vi "Generator DC Sweep Manager.vi"(8 "error in (no error)":errorcluster, 10 "sweep index":i32=-1, 11 "LockinDAQ":refnum<class "LockinDAQ.lvclass">) -> (0 "error out":errorcluster, 1 "Start (V)":dbl[](array[numeric]), 2 "End (V)":dbl[](array[numeric]), 3 "LockinDAQ out":refnum<class "LockinDAQ.lvclass">)   [LabVIEW 2016, in "LockinDAQ.lvclass"]
uses:
  LockinDAQ.lvclass
  LockinDAQ.lvclass/LockinDAQ.ctl
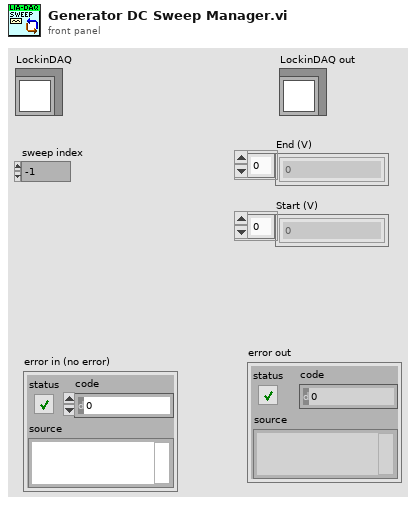
[diagram p1: front panel]
types:
  T1 = typedef "LockinDAQ.lvclass/AO-cluster.ctl" = cluster{"Ch":i32[], "Amp (V)":dbl[], "DC (V)":dbl[], "f (Hz)":dbl[], "Phase (°)":dbl[], "Function":T2[], "Sweep?":bool[]}
  T2 = typedef "LockinDAQ.lvclass/Function-enum.ctl" = enum16{"Sine", "Triangle", "Square", "Sawtooth"}
  T3 = typedef "LockinDAQ.lvclass/Sweep Configuration--Cluster.ctl" = cluster{"Sweep Type":enum16{"sweepLockin", "sweepIV"}, "Sweep Lockin Time (s)":dbl, "Sweep IV Step (V)":dbl, "Initial Wait Time (s)":dbl, "Sweep Channel":i32[], "Sweep Start (V)":dbl[], "Sweep End (V)":dbl[], "Return to Start":bool}
  T4 = typedef "LockinDAQ.lvclass/Sampling.ctl" = cluster{"Fs":dbl, "#s":i32}
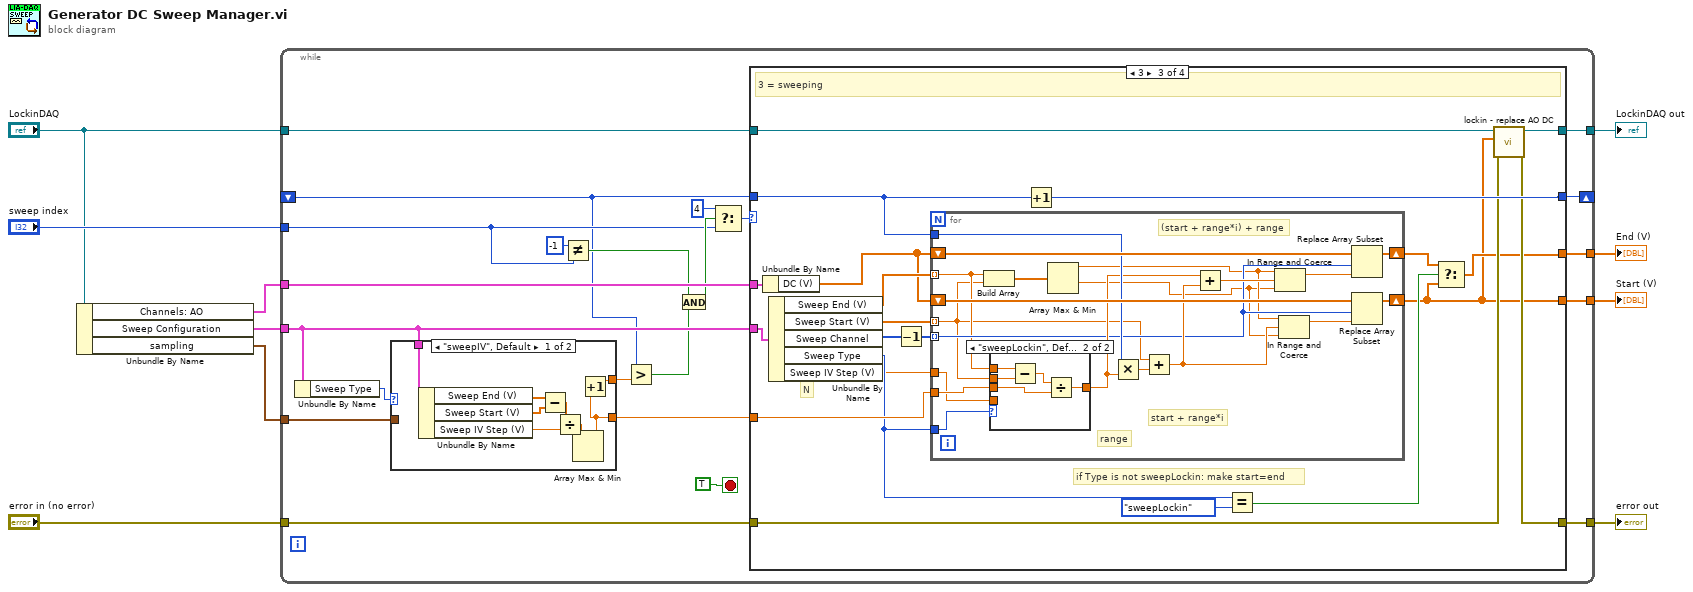
[diagram p0: block diagram]
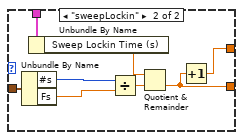
[diagram p2: hidden frame]
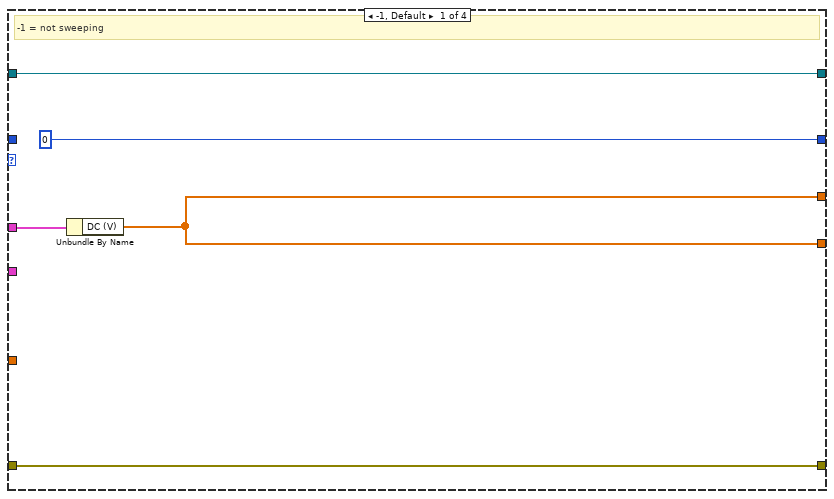
[diagram p3: hidden frame]
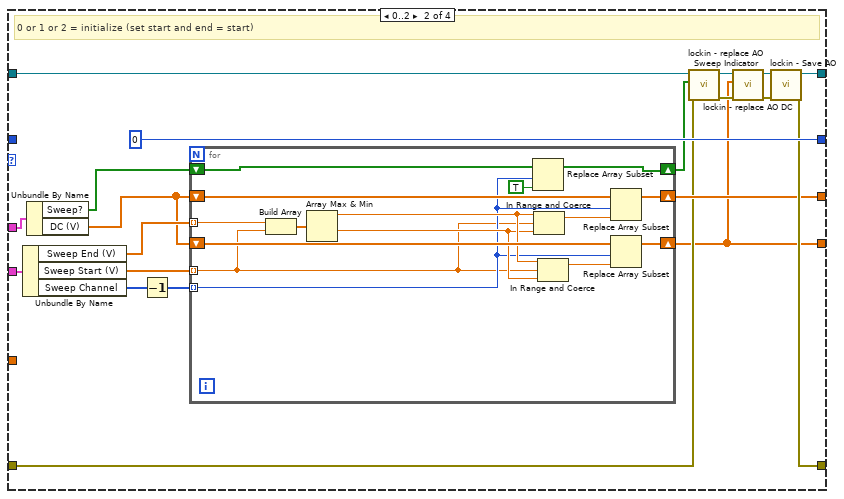
[diagram p4: hidden frame]
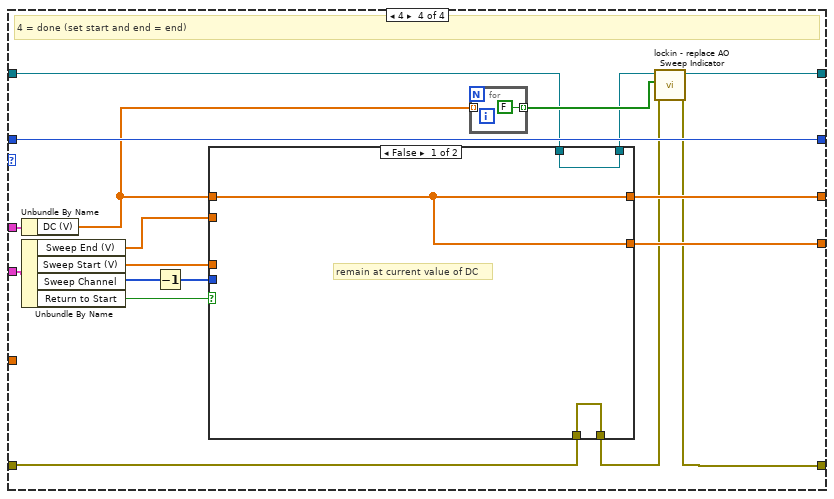
[diagram p6: hidden frame]
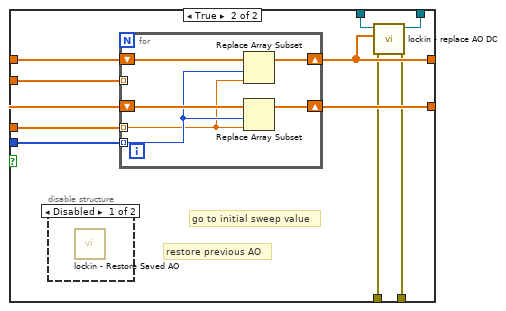
[diagram p7: hidden frame]
diagram:
  n1 = Unbundle By Name("LockinDAQ") -> ("Channels: AO"=w6:T1, "Sweep Configuration"=w7:T3, "sampling"=w8:T4)
  n2 = while {
    tunnel: w6 -> [w32]
    tunnel: [w17] -> w9
    tunnel: [w31] -> w10
    tunnel: w7 -> [w15]
    tunnel: "sweep index" -> [w16]
    tunnel: w8 -> [w28]
    shift-right: [w30] -> _
    shift-left: _ -> [w12]
    tunnel: [w21] -> w4
    tunnel: "LockinDAQ" -> [w20]
    tunnel: "error in (no error)" -> [w19]
    tunnel: [w18] -> w1
    stop <- TRUE stop-if-true
    n3 = Unbundle By Name(w15) -> ("Sweep Type"=w14:enum16{"sweepLockin", "sweepIV"})
    n4 = case shown="\"sweepIV\", Default" w14 {
      tunnel: w28 -> [_ w44]
      tunnel: [w34 w43] -> w25
      tunnel: w15 -> [w40 w42]
      tunnel: [w33 w41] -> w13
      frame "sweepIV", Default {
        n5 = Unbundle By Name(w40) -> ("Sweep End (V)"=w39:dbl[], "Sweep Start (V)"=w38:dbl[], "Sweep IV Step (V)"=w36:dbl)
        n6 = Subtract(x=w39, y=w38) -> (x-y=w37:dbl[])
        n7 = Divide(x=w37, y=w36) -> (x/y=w35:dbl[])
        n8 = Array Max & Min(array=w35) -> (max value=w34:dbl)  [unwired: 3 out]
        n9 = Increment(x=w34) -> (x+1=w33:dbl)
      }
      frame "sweepLockin" {
        n10 = Unbundle By Name(w44) -> ("#s"=w45:i32, "Fs"=w48:dbl)
        n11 = Unbundle By Name(w42) -> ("Sweep Lockin Time (s)"=w47:dbl)
        n12 = Divide(x=w45, y=w48) -> (x/y=w46:dbl)
        n13 = Quotient & Remainder(x=w47, y=w46) -> (floor(x/y)=w43:dbl)  [unwired: 1 out]
        n14 = Increment(x=w43) -> (x+1=w41:dbl)
      }
    }
    n15 = Not Equal?(x=-1, y=w16) -> (x != y?=w22:bool)
    n16 = Greater?(x=w12, y=w13) -> (0:w11:bool)
    n17 = And(x=w22, y=w11) -> (x .and. y?=w23:bool)
    n18 = Select(t=4, s=w23, f=w16) -> (s? t:f=w26:i32)
    n19 = case shown="3" w26 {
      tunnel: w32 -> [w53 w73 w109 w153]
      tunnel: [w52 w54 w91 w151] -> w31
      tunnel: w15 -> [_ w69 w105 w148]
      tunnel: [0 0 w101 w146] -> w30
      tunnel: w12 -> [_ _ w102 w146]
      tunnel: w25 -> [_ _ w100 _]
      tunnel: [w50 w65 w96 w137] -> w21
      tunnel: w20 -> [w50 w61 w98 w141]
      tunnel: w19 -> [w49 w57 w99 w139]
      tunnel: [w49 w64 w97 w136] -> w18
      tunnel: [w52 w62 w92 w145] -> w17
      frame -1, Default {
        # "-1 = not sweeping"
        n20 = Unbundle By Name(w53) -> ("DC (V)"=w52:dbl[])
      }
      frame 0..2 {
        # "0 or 1 or 2 = initialize (set start and end = start)"
        n21 = Unbundle By Name(w69) -> ("Sweep End (V)"=w70:dbl[], "Sweep Start (V)"=w71:dbl[], "Sweep Channel"=w72:i32[])
        n22 = Unbundle By Name(w73) -> ("Sweep?"=w59:bool[], "DC (V)"=w67:dbl[])
        n23 = Decrement(x=w72) -> (x-1=w68:i32[])
        n24 = for {
          shift-right: [w87] -> w62
          shift-left: w67 -> [w88]
          shift-right: [w85] -> w54
          shift-left: w67 -> [w86]
          tunnel: w71 -> [w74] mode=indexing
          tunnel: w70 -> [w81] mode=indexing
          tunnel: w68 -> [w76] mode=indexing
          shift-right: [w77] -> w55
          shift-left: w59 -> [w78]
          n25 = Build Array(w81, w74) -> (w82:dbl[])
          n26 = Array Max & Min(array=w82) -> (max value=w80:dbl, min value=w79:dbl)  [unwired: 2 out]
          n27 = Replace Array Subset(array=w78, new element=TRUE ("new element/subarray"), index=w76) -> (w77:bool[])
          n28 = In Range and Coerce(upper limit=w80, x=w74, lower limit=w79) -> (coerced(x)=w84:dbl)  [unwired: 1 out]
          n29 = In Range and Coerce(upper limit=w80, x=w74, lower limit=w79) -> (coerced(x)=w83:dbl)  [unwired: 1 out]
          n30 = Replace Array Subset(array=w88, new element=w84, index=w76) -> (w87:dbl[])
          n31 = Replace Array Subset(array=w86, new element=w83, index=w76) -> (w85:dbl[])
        }
        n32 = call "lockin - replace AO Sweep Indicator.vi"("error in (no error)"=w57, "Channels: AO.Sweep?"=w55, "LockinDAQ"=w61) -> ("error out"=w58:errorcluster, "LockinDAQ out"=w60:refnum<class "LockinDAQ.lvclass">)  [unwired: 7 in]
        n33 = call "lockin - replace AO DC.vi"("error in (no error)"=w58, "AO.DC (V)"=w54, "LockinDAQ"=w60) -> ("error out"=w56:errorcluster, "LockinDAQ out"=w63:refnum<class "LockinDAQ.lvclass">)  [unwired: 7 in]
        n34 = call "lockin - Save AO.vi"("error in (no error)"=w56, "LockinDAQ"=w63) -> ("error out"=w64:errorcluster, "LockinDAQ out"=w65:refnum<class "LockinDAQ.lvclass">)  [unwired: 8 in]
      }
      frame 3 {
        # "if Type is not sweepLockin: make start=end"
        # "N"
        # "3 = sweeping"
        n35 = Unbundle By Name(w109) -> ("DC (V)"=w103:dbl[])
        n36 = Unbundle By Name(w105) -> ("Sweep End (V)"=w106:dbl[], "Sweep Start (V)"=w107:dbl[], "Sweep Channel"=w108:i32[], "Sweep Type"=w90:enum16{"sweepLockin", "sweepIV"}, "Sweep IV Step (V)"=w89:dbl)
        n37 = Decrement(x=w108) -> (x-1=w104:i32[])
        n38 = for {
          shift-right: [w128] -> w93
          shift-left: w103 -> [w129]
          shift-right: [w126] -> w91
          shift-left: w103 -> [w127]
          tunnel: w107 -> [w115] mode=indexing
          tunnel: w106 -> [w116] mode=indexing
          tunnel: w104 -> [w117] mode=indexing
          tunnel: w102 -> [w123]
          tunnel: w100 -> [w125]
          tunnel: w90 -> [w111]
          tunnel: w89 -> [w110]
          # "(start + range*i) + range"
          # "start + range*i"
          # "range"
          n39 = Build Array(w116, w115) -> (w114:dbl[])
          n40 = case shown="\"sweepLockin\", Default" w111 {
            tunnel: w125 -> [_ w135]
            tunnel: [w130 w133] -> w122
            tunnel: w116 -> [_ w132]
            tunnel: w115 -> [_ w131]
            tunnel: w110 -> [w130 _]
            frame "sweepIV" {
            }
            frame "sweepLockin", Default {
              n41 = Subtract(x=w132, y=w131) -> (x-y=w134:dbl)
              n42 = Divide(x=w134, y=w135) -> (x/y=w133:dbl)
            }
          }
          n43 = Array Max & Min(array=w114) -> (max value=w113:dbl, min value=w112:dbl)  [unwired: 2 out]
          n44 = Multiply(x=w123, y=w122) -> (x*y=w124:dbl)
          n45 = Add(x=w115, y=w124) -> (x+y=w118:dbl)
          n46 = Add(x=w122, y=w118) -> (x+y=w121:dbl)
          n47 = In Range and Coerce(upper limit=w113, x=w121, lower limit=w112) -> (coerced(x)=w120:dbl)  [unwired: 1 out]
          n48 = In Range and Coerce(upper limit=w113, x=w118, lower limit=w112) -> (coerced(x)=w119:dbl)  [unwired: 1 out]
          n49 = Replace Array Subset(array=w129, new element=w120, index=w117) -> (w128:dbl[])
          n50 = Replace Array Subset(array=w127, new element=w119, index=w117) -> (w126:dbl[])
        }
        n51 = Increment(x=w102) -> (x+1=w101:i32)
        n52 = Equal?(x=w90, y=enum16{"sweepLockin", "sweepIV"}."sweepLockin" ("Type")) -> (x = y?=w94:bool)
        n53 = Select(t=w93, s=w94, f=w91) -> (s? t:f=w92:dbl[])
        n54 = call "lockin - replace AO DC.vi"("error in (no error)"=w99, "AO.DC (V)"=w91, "LockinDAQ"=w98) -> ("error out"=w97:errorcluster, "LockinDAQ out"=w96:refnum<class "LockinDAQ.lvclass">)  [unwired: 7 in]
      }
      frame 4 {
        # "4 = done (set start and end = end)"
        n55 = Unbundle By Name(w153) -> ("DC (V)"=w143:dbl[])
        n56 = Unbundle By Name(w148) -> ("Sweep End (V)"=w149:dbl[], "Sweep Start (V)"=w150:dbl[], "Sweep Channel"=w152:i32[], "Return to Start"=w144:bool)
        n57 = Decrement(x=w152) -> (x-1=w147:i32[])
        n58 = case shown="False" w144 {
          tunnel: [w157 w167] -> w151
          tunnel: w150 -> [_ w166]
          tunnel: w149 -> [_ w165]
          tunnel: w147 -> [_ w164]
          tunnel: w143 -> [w157 w163]
          tunnel: [w157 w160] -> w145
          tunnel: w141 -> [w156 w162]
          tunnel: [w156 w161] -> w140
          tunnel: w139 -> [w155 w159]
          tunnel: [w155 w158] -> w138
          frame False {
            # "remain at current value of DC"
          }
          frame True {
            # "restore previous AO"
            # "go to initial sweep value"
            n59 = disable-structure shown="Disabled" {
              frame Disabled {
                n60 = call "lockin - Restore Saved AO.vi"() -> ()  [unwired: 10 in, 2 out]
              }
              frame Enabled {
              }
            }
            n61 = for {
              shift-right: [w172] -> w160
              shift-left: w163 -> [w173]
              shift-right: [w170] -> w167
              shift-left: w163 -> [w171]
              tunnel: w166 -> [w168] mode=indexing
              tunnel: w165 -> [_] mode=indexing
              tunnel: w164 -> [w169] mode=indexing
              n62 = Replace Array Subset(array=w173, new element=w168, index=w169) -> (w172:dbl[])
              n63 = Replace Array Subset(array=w171, new element=w168, index=w169) -> (w170:dbl[])
            }
            n64 = call "lockin - replace AO DC.vi"("error in (no error)"=w159, "AO.DC (V)"=w160, "LockinDAQ"=w162) -> ("error out"=w158:errorcluster, "LockinDAQ out"=w161:refnum<class "LockinDAQ.lvclass">)  [unwired: 7 in]
          }
        }
        n65 = for {
          tunnel: w143 -> [_] mode=indexing
          tunnel: [FALSE] -> w142 mode=indexing
        }
        n66 = call "lockin - replace AO Sweep Indicator.vi"("error in (no error)"=w138, "Channels: AO.Sweep?"=w142, "LockinDAQ"=w140) -> ("error out"=w136:errorcluster, "LockinDAQ out"=w137:refnum<class "LockinDAQ.lvclass">)  [unwired: 7 in]
      }
    }
  }
  "Start (V)" <- w10
  "End (V)" <- w9
  "LockinDAQ out" <- w4
  "error out" <- w1
